vi "UI_(02)_Unlock.vi"(3 "error in (no error)":errorcluster, 4 "Settings cluster in":T1={"Defaults"={"Default User"=0.0, "VISA Resource Name "="", "Histogram parameters"={"max"=300.0, "min"=0.0, "# bins"=10, "threshold"=8.0, "thr. type"=enum."higher accepted"}}, "Recording and saving"={"Researcher name"="", "Name prefix"="", "Data post-processing"={"Filter type"=enum."Savitzky-Golay", "Length"=31, "Order"=3}, "Stop at"=0.0, "\"Stop at\" enabled"=FALSE, "Default save folder path"=path "", "Acquisition FPS"=enum."Max"}, "Geometry"={"Sensor board size"=enum."", "Bridge swap"=FALSE, "Twisted neck"=FALSE, "Bridge H. offset"=0.0, "Bridge V. offset"=0.0, "Magnets orientation"=0.0, "Cage type"=0, "Cage parameters"={"Round"=variant(i16 0), "Square"=variant(u16 0), "Donut-maze"=variant(u16 0), "T-maze"=variant(u8 0), "Sociability-maze"=variant(u8 0)}}, "IO parameters"={"IO general config."=0, "IO 1 configuration"=0, "IO 2 configuration"=0, "IO 3 configuration"=0, "IO 4 configuration"=0, "Activate ext. RS-232"=0, "IO inversion config."=0, "Sync capability"=1}, "Conditions presets array"=[{"Enabled"=FALSE, "Name"="", "Specifier(s)"=[], "Response"={"Response type"=enum."Air puff", "TTL port"=enum."Port 1", "TTL pulse length, ms"=0.0}, "Has been set"=FALSE}, {"Enabled"=FALSE, "Name"="", "Specifier(s)"=[], "Response"={"Response type"=enum."Air puff", "TTL port"=enum."Port 1", "TTL pulse length, ms"=0.0}, "Has been set"=FALSE}, {"Enabled"=FALSE, "Name"="", "Specifier(s)"=[], "Response"={"Response type"=enum."Air puff", "TTL port"=enum."Port 1", "TTL pulse length, ms"=0.0}, "Has been set"=FALSE}, {"Enabled"=FALSE, "Name"="", "Specifier(s)"=[], "Response"={"Response type"=enum."Air puff", "TTL port"=enum."Port 1", "TTL pulse length, ms"=0.0}, "Has been set"=FALSE}, {"Enabled"=FALSE, "Name"="", "Specifier(s)"=[], "Response"={"Response type"=enum."Air puff", "TTL port"=enum."Port 1", "TTL pulse length, ms"=0.0}, "Has been set"=FALSE}, {"Enabled"=FALSE, "Name"="", "Specifier(s)"=[], "Response"={"Response type"=enum."Air puff", "TTL port"=enum."Port 1", "TTL pulse length, ms"=0.0}, "Has been set"=FALSE}, {"Enabled"=FALSE, "Name"="", "Specifier(s)"=[], "Response"={"Response type"=enum."Air puff", "TTL port"=enum."Port 1", "TTL pulse length, ms"=0.0}, "Has been set"=FALSE}, {"Enabled"=FALSE, "Name"="", "Specifier(s)"=[], "Response"={"Response type"=enum."Air puff", "TTL port"=enum."Port 1", "TTL pulse length, ms"=0.0}, "Has been set"=FALSE}, {"Enabled"=FALSE, "Name"="", "Specifier(s)"=[], "Response"={"Response type"=enum."Air puff", "TTL port"=enum."Port 1", "TTL pulse length, ms"=0.0}, "Has been set"=FALSE}, {"Enabled"=FALSE, "Name"="", "Specifier(s)"=[], "Response"={"Response type"=enum."Air puff", "TTL port"=enum."Port 1", "TTL pulse length, ms"=0.0}, "Has been set"=FALSE}, {"Enabled"=FALSE, "Name"="", "Specifier(s)"=[], "Response"={"Response type"=enum."Air puff", "TTL port"=enum."Port 1", "TTL pulse length, ms"=0.0}, "Has been set"=FALSE}, {"Enabled"=FALSE, "Name"="", "Specifier(s)"=[], "Response"={"Response type"=enum."Air puff", "TTL port"=enum."Port 1", "TTL pulse length, ms"=0.0}, "Has been set"=FALSE}, {"Enabled"=FALSE, "Name"="", "Specifier(s)"=[], "Response"={"Response type"=enum."Air puff", "TTL port"=enum."Port 1", "TTL pulse length, ms"=0.0}, "Has been set"=FALSE}, {"Enabled"=FALSE, "Name"="", "Specifier(s)"=[], "Response"={"Response type"=enum."Air puff", "TTL port"=enum."Port 1", "TTL pulse length, ms"=0.0}, "Has been set"=FALSE}], "Calibration parameters"={"Timing calibration sw/hw"=1.0, "True FPS"=80.0, "True frame time, s"=80.0, "Disp. calibration info"=[]}, "Settings loaded OK"=FALSE} {"Calibration parameters"."True frame time, s" format="%.10g"; "Calibration parameters"."Disp. calibration info"."Speed, µl per ms" format="%.3g"; "Calibration parameters"."True FPS" format="%.10g"; "Calibration parameters"."Timing calibration sw/hw" format="%.10g"; "Conditions presets array"."Specifier(s)"."Validity criteria(s)"."Validity value" min=0.0 step=0.1 format="%.2g"; "Conditions presets array"."Specifier(s)"."Value" step=1.0 format="%#.2g"; "Recording and saving"."Data post-processing"."Order" min=3 max=11 step=2; "Recording and saving"."Data post-processing"."Length" min=5 max=301 step=2; "Geometry"."Cage type" items=["Round", "Square", "Donut-maze", "T-maze", "Sociability maze", ""]}, 5 "All references in":T21) -> (0 "error out":errorcluster, 1 "Settings cluster out":T1={"Defaults"={"Default User"=0.0, "VISA Resource Name "="", "Histogram parameters"={"max"=300.0, "min"=0.0, "# bins"=10, "threshold"=8.0, "thr. type"=enum."higher accepted"}}, "Recording and saving"={"Researcher name"="", "Name prefix"="", "Data post-processing"={"Filter type"=enum."Savitzky-Golay", "Length"=31, "Order"=3}, "Stop at"=0.0, "\"Stop at\" enabled"=FALSE, "Default save folder path"=path "", "Acquisition FPS"=enum."Max"}, "Geometry"={"Sensor board size"=enum."", "Bridge swap"=FALSE, "Twisted neck"=FALSE, "Bridge H. offset"=0.0, "Bridge V. offset"=0.0, "Magnets orientation"=0.0, "Cage type"=0, "Cage parameters"={"Round"=variant(i16 0), "Square"=variant(u16 0), "Donut-maze"=variant(u16 0), "T-maze"=variant(u8 0), "Sociability-maze"=variant(u8 0)}}, "IO parameters"={"IO general config."=0, "IO 1 configuration"=0, "IO 2 configuration"=0, "IO 3 configuration"=0, "IO 4 configuration"=0, "Activate ext. RS-232"=0, "IO inversion config."=0, "Sync capability"=1}, "Conditions presets array"=[{"Enabled"=FALSE, "Name"="", "Specifier(s)"=[], "Response"={"Response type"=enum."Air puff", "TTL port"=enum."Port 1", "TTL pulse length, ms"=0.0}, "Has been set"=FALSE}, {"Enabled"=FALSE, "Name"="", "Specifier(s)"=[], "Response"={"Response type"=enum."Air puff", "TTL port"=enum."Port 1", "TTL pulse length, ms"=0.0}, "Has been set"=FALSE}, {"Enabled"=FALSE, "Name"="", "Specifier(s)"=[], "Response"={"Response type"=enum."Air puff", "TTL port"=enum."Port 1", "TTL pulse length, ms"=0.0}, "Has been set"=FALSE}, {"Enabled"=FALSE, "Name"="", "Specifier(s)"=[], "Response"={"Response type"=enum."Air puff", "TTL port"=enum."Port 1", "TTL pulse length, ms"=0.0}, "Has been set"=FALSE}, {"Enabled"=FALSE, "Name"="", "Specifier(s)"=[], "Response"={"Response type"=enum."Air puff", "TTL port"=enum."Port 1", "TTL pulse length, ms"=0.0}, "Has been set"=FALSE}, {"Enabled"=FALSE, "Name"="", "Specifier(s)"=[], "Response"={"Response type"=enum."Air puff", "TTL port"=enum."Port 1", "TTL pulse length, ms"=0.0}, "Has been set"=FALSE}, {"Enabled"=FALSE, "Name"="", "Specifier(s)"=[], "Response"={"Response type"=enum."Air puff", "TTL port"=enum."Port 1", "TTL pulse length, ms"=0.0}, "Has been set"=FALSE}, {"Enabled"=FALSE, "Name"="", "Specifier(s)"=[], "Response"={"Response type"=enum."Air puff", "TTL port"=enum."Port 1", "TTL pulse length, ms"=0.0}, "Has been set"=FALSE}, {"Enabled"=FALSE, "Name"="", "Specifier(s)"=[], "Response"={"Response type"=enum."Air puff", "TTL port"=enum."Port 1", "TTL pulse length, ms"=0.0}, "Has been set"=FALSE}, {"Enabled"=FALSE, "Name"="", "Specifier(s)"=[], "Response"={"Response type"=enum."Air puff", "TTL port"=enum."Port 1", "TTL pulse length, ms"=0.0}, "Has been set"=FALSE}, {"Enabled"=FALSE, "Name"="", "Specifier(s)"=[], "Response"={"Response type"=enum."Air puff", "TTL port"=enum."Port 1", "TTL pulse length, ms"=0.0}, "Has been set"=FALSE}, {"Enabled"=FALSE, "Name"="", "Specifier(s)"=[], "Response"={"Response type"=enum."Air puff", "TTL port"=enum."Port 1", "TTL pulse length, ms"=0.0}, "Has been set"=FALSE}, {"Enabled"=FALSE, "Name"="", "Specifier(s)"=[], "Response"={"Response type"=enum."Air puff", "TTL port"=enum."Port 1", "TTL pulse length, ms"=0.0}, "Has been set"=FALSE}, {"Enabled"=FALSE, "Name"="", "Specifier(s)"=[], "Response"={"Response type"=enum."Air puff", "TTL port"=enum."Port 1", "TTL pulse length, ms"=0.0}, "Has been set"=FALSE}], "Calibration parameters"={"Timing calibration sw/hw"=1.0, "True FPS"=80.0, "True frame time, s"=80.0, "Disp. calibration info"=[]}, "Settings loaded OK"=FALSE} {"Calibration parameters"."True frame time, s" format="%.10g"; "Calibration parameters"."Disp. calibration info"."Speed, µl per ms" format="%.3g"; "Calibration parameters"."True FPS" format="%.10g"; "Calibration parameters"."Timing calibration sw/hw" format="%.10g"; "Conditions presets array"."Specifier(s)"."Validity criteria(s)"."Validity value" min=0.0 step=0.1 format="%.2g"; "Conditions presets array"."Specifier(s)"."Value" step=1.0 format="%#.2g"; "Recording and saving"."Data post-processing"."Order" min=3 max=11 step=2; "Recording and saving"."Data post-processing"."Length" min=5 max=301 step=2; "Geometry"."Cage type" items=["Round", "Square", "Donut-maze", "T-maze", "Sociability maze", ""]}, 2 "All references out":T21)   [LabVIEW 2018, in "Tracker.lvlib"]
uses:
  Tracker.lvlib
  Controls/CTL_All_References.ctl
  Controls/CTL_Controls_References.ctl
  Controls/CTL_Indicators_References.ctl
  Common/Typedefs/CTL_Panes_and_VIs_References.ctl
  Controls/CTL_Histogram_Properties.ctl
  <vilib>/Utility/miscctls.llb/LVRangeTypeDef.ctl
  Controls/CTL_Settings_cluster.ctl
  Controls/CTL_Histogram_parameters.ctl
  Controls/CTL_Filter_selector.ctl
  Controls/CTL_Acquisition_speed_selector.ctl
  Common/Typedefs/CTL_Segmented_plot_parameters_2.ctl
  Libraries/Cage Diagram/Typedefs/CTL_Cage_type.ctl
  Controls/CTL_Cage_all_segmentation_params_set.ctl
  Controls/CTL_IO_params_cluster.ctl
  Controls/CTL_Conditions_Array.ctl
  Controls/CTL_Conditions_Cluster.ctl
  Controls/CTL_Condition_type.ctl
  Controls/CTL_Comparison_type.ctl
  Controls/CTL_Validity_check_criteria.ctl
  Controls/CTL_Response_info.ctl
  Controls/CTL_Condition_response_type.ctl
  Controls/CTL_Reponse_port_info.ctl
  Controls/CTL_Calibration_parameters.ctl
  Controls/CTL_Dispenser_calibration_info.ctl
  Common/Typedefs/CTL_Segmented_plot_parameters_2_(round_d1).ctl
  <vilib>/Utility/error.llb/Error Cluster From Error Code.vi
  <vilib>/ErrorRing/Error Ring.xnode
  Common_Resources.lvlib
  Libraries/Cage Diagram/Cage Diagram.lvlib
panel:
  in  "Histogram initialization cluster":T19={"X Scale.Range"={"Minimum"=0.0, "Maximum"=13.0, "Increment"=1.0, "Minor Increment"=1.0, "Start"=0.0}, "Caption.Text"="Zone preference (normalized)", "X Scale.Offset and Multiplier:Multiplier"=1.0, "X Scale.Offset and Multiplier:Offset"=0.0, "X Scale.Scale Fit"=2, "X Scale.Display Format:Precision"=0, "Y Scale.Mapping Mode"=0, "Zones preference empty initialized array"=[0, 0, 0, 0, 0, 0, 0, 0, 0, 0, 0, 0, 0, 0], "Plot.Fill/Point Color"=15790320}
  out "Panes references":T24
  out "Controls references params":string[][](array[string])
  out "Indicators references params":string[][](array[string])
  out "Indicators references":T23
  out "Controls references":T22
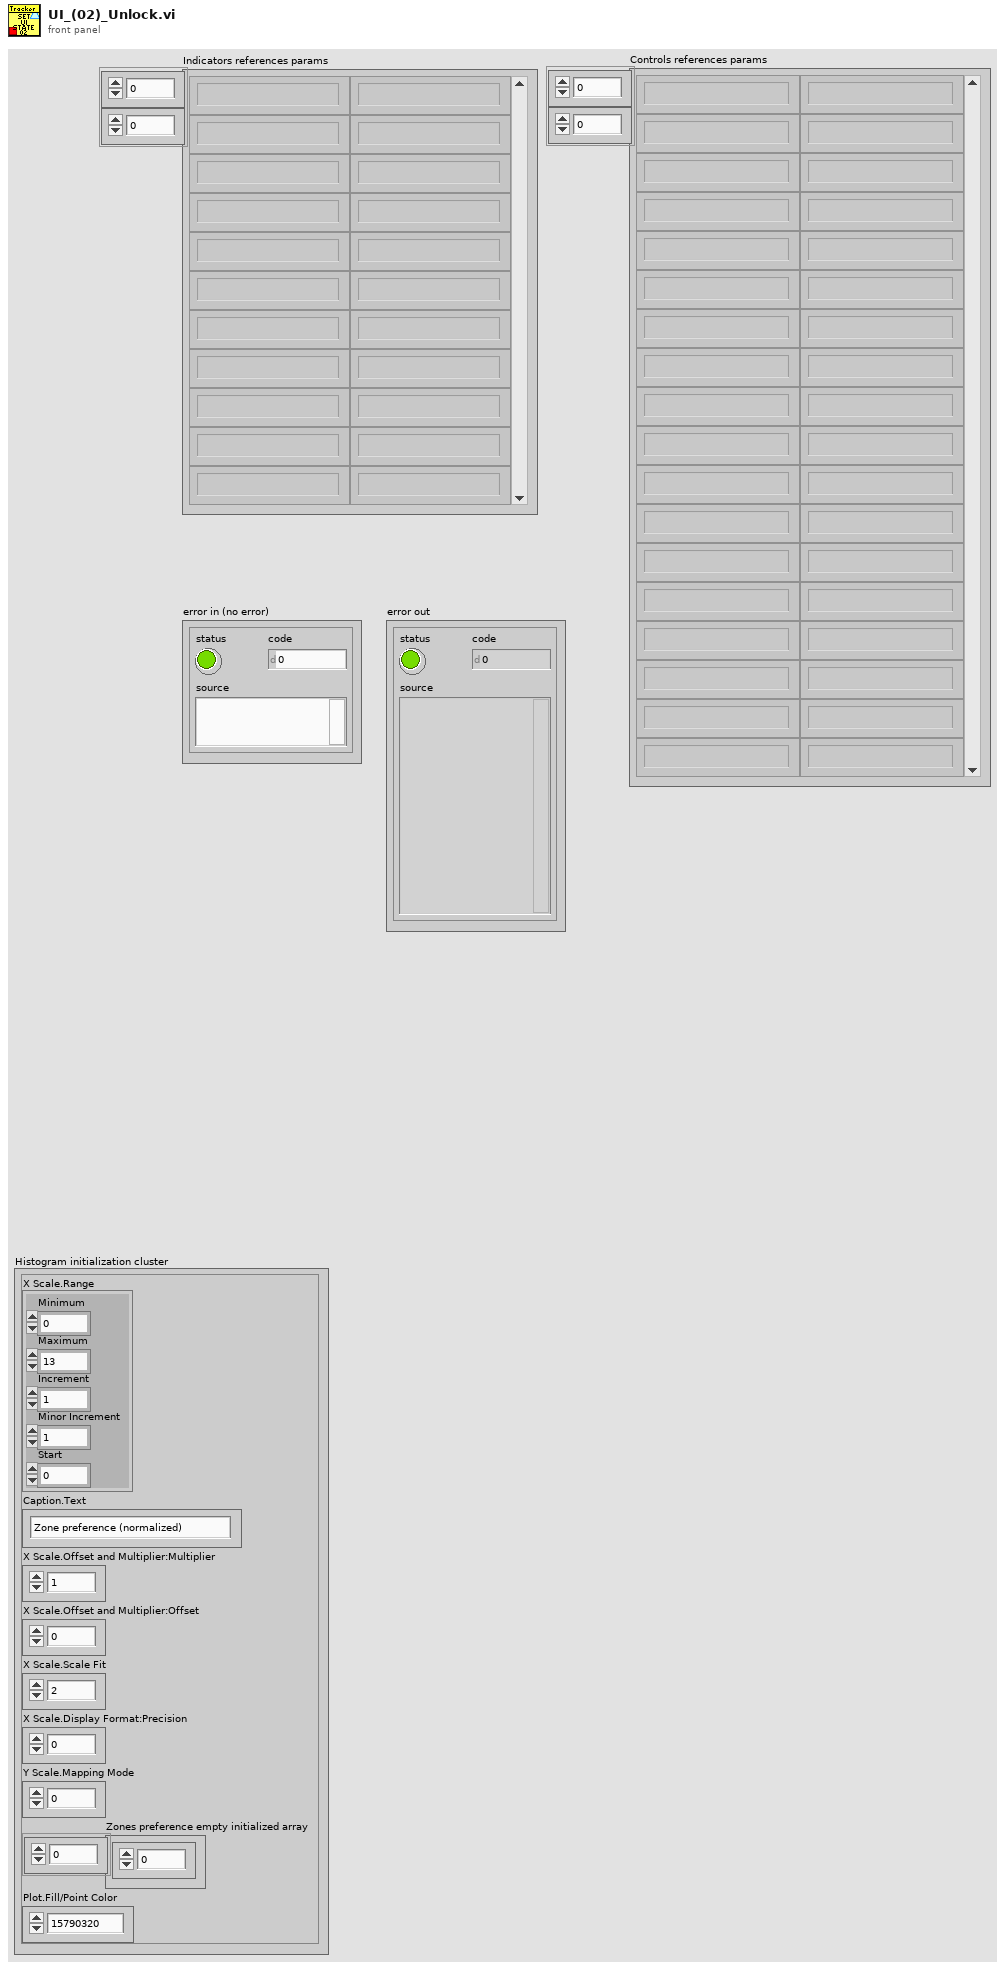
[diagram p1: front panel]
types:
  T1 = typedef "Common_Resources.lvlib/CTL_Settings_cluster.ctl" = cluster{"Defaults":cluster{"Default User":dbl, "VISA Resource Name ":string, "Histogram parameters":T2}, "Recording and saving":cluster{"Researcher name":string, "Name prefix":string, "Data post-processing":T3, "Stop at":dbl, "\"Stop at\" enabled":bool, "Default save folder path":path, "Acquisition FPS":T4}, "Geometry":T5, "IO parameters":T8, "Conditions presets array":T9, "Calibration parameters":T17, "Settings loaded OK":bool}
  T2 = typedef "Common_Resources.lvlib/CTL_Histogram_parameters.ctl" = cluster{"max":dbl, "min":dbl, "# bins":i32, "threshold":dbl, "thr. type":enum16{"higher accepted", "lower accepted"}}
  T3 = typedef "Common_Resources.lvlib/CTL_Filter_selector.ctl" = cluster{"Filter type":enum16{"None", "Savitzky-Golay"}, "Length":i32, "Order":i32}
  T4 = typedef "Common_Resources.lvlib/CTL_Acquisition_speed_selector.ctl" = enum16{"Max", "Optimal", "Eco"}
  T5 = typedef "Common_Resources.lvlib/CTL_Segmented_plot_parameters_2.ctl" = cluster{"Sensor board size":enum16{"", "Large"}, "Bridge swap":bool, "Twisted neck":bool, "Bridge H. offset":sgl, "Bridge V. offset":sgl, "Magnets orientation":sgl, "Cage type":T6, "Cage parameters":T7}
  T6 = typedef "Cage Diagram.lvlib/CTL_Cage_type.ctl" = u16
  T7 = typedef "Common_Resources.lvlib/CTL_Cage_all_segmentation_params_set.ctl" = cluster{"Round":variant, "Square":variant, "Donut-maze":variant, "T-maze":variant, "Sociability-maze":variant}
  T8 = typedef "Common_Resources.lvlib/CTL_IO_params_cluster.ctl" = cluster{"IO general config.":u16, "IO 1 configuration":u16, "IO 2 configuration":u16, "IO 3 configuration":u16, "IO 4 configuration":u16, "Activate ext. RS-232":u16, "IO inversion config.":u16, "Sync capability":u8}
  T9 = typedef "Common_Resources.lvlib/CTL_Conditions_Array.ctl" = T10[]
  T10 = typedef "Common_Resources.lvlib/CTL_Conditions_Cluster.ctl" = cluster{"Enabled":bool, "Name":string, "Specifier(s)":cluster{"Specifier enabled":bool, "Condition type":T11, "Comparison type":T12, "Value":dbl, "Validity criteria(s)":cluster{"V. check enabled":bool, "Criteria":T13, "Validity value":dbl}[]}[], "Response":T14, "Has been set":bool}
  T11 = typedef "Common_Resources.lvlib/CTL_Condition_type.ctl" = enum16{"Speed", "Zone", "Angle to wall"}
  T12 = typedef "Common_Resources.lvlib/CTL_Comparison_type.ctl" = enum16{"Less", "Less or Equal", "Equal", "Greater or Equal", "Greater", "Not Equal"}
  T13 = typedef "Common_Resources.lvlib/CTL_Validity_check_criteria.ctl" = enum16{"Running bout (seconds)", "Running bout (meters)"}
  T14 = typedef "Common_Resources.lvlib/CTL_Response_info.ctl" = cluster{"Response type":T15, "TTL port":T16, "TTL pulse length, ms":dbl}
  T15 = typedef "Common_Resources.lvlib/CTL_Condition_response_type.ctl" = enum16{"None", "Air puff", "Liquid reward", "TTL pulse", "TTL pulse (ubr)", "TTL signal"}
  T16 = typedef "Common_Resources.lvlib/CTL_Reponse_port_info.ctl" = enum16{"Port 1", "Port 2", "Port 3", "Port 4"}
  T17 = typedef "Common_Resources.lvlib/CTL_Calibration_parameters.ctl" = cluster{"Timing calibration sw/hw":dbl, "True FPS":dbl, "True frame time, s":dbl, "Disp. calibration info":T18}
  T18 = typedef "Common_Resources.lvlib/CTL_Dispenser_calibration_info.ctl" = cluster{"Channel":u8, "Speed, µl per ms":dbl}[]
  T19 = typedef "Common_Resources.lvlib/CTL_Histogram_Properties.ctl" = cluster{"X Scale.Range":T20, "Caption.Text":string, "X Scale.Offset and Multiplier:Multiplier":dbl, "X Scale.Offset and Multiplier:Offset":dbl, "X Scale.Scale Fit":u8, "X Scale.Display Format:Precision":u8, "Y Scale.Mapping Mode":u8, "Zones preference empty initialized array":i32[], "Plot.Fill/Point Color":u32}
  T20 = typedef "LVRangeTypeDef.ctl" = cluster{"Minimum":dbl, "Maximum":dbl, "Increment":dbl, "Minor Increment":dbl, "Start":dbl}
  T21 = typedef "Common_Resources.lvlib/CTL_All_References.ctl" = cluster{"Controls references":T22, "Indicators references":T23, "Service references":T24}
  T22 = typedef "Common_Resources.lvlib/CTL_Controls_References.ctl" = cluster{"Check HW connection":refnum<vi>, "Save settings":refnum<vi>, "Reset zones":refnum<vi>, "Reset stimuli":refnum<vi>, "Record/Stop":refnum<vi>, "Reset barplot":refnum<vi>, "Multiplyer of chart RX":refnum<vi>, "Show zones":refnum<vi>, "Show magnets":refnum<vi>, "Show heatmap":refnum<vi>, "Show full track":refnum<vi>, "Open File":refnum<vi>, "Play/Pause":refnum<vi>, "Trace, s":refnum<vi>, "Playback speed":refnum<vi>, "Timeline":refnum<vi>, "By Zone stim. setup":refnum<vi>, "Set/Rec and Analyse Tab":refnum<vi>, "Cage radial segmentation":refnum<vi>, "Set IO config":refnum<vi>, "Rainbow (time)":refnum<vi>, "Rainbow (speed)":refnum<vi>, "Add Reward":refnum<vi>, "Modify Reward":refnum<vi>, "Delete Reward":refnum<vi>, "Speed threshold, mm/s":refnum<vi>, "Start Over":refnum<vi>}
  T23 = typedef "Common_Resources.lvlib/CTL_Indicators_References.ctl" = cluster{"HW info":refnum<vi>, "Port":refnum<vi>, "Ready":refnum<vi>, "IO status indicator":refnum<vi>, "Current Time":refnum<vi>, "Record timestamp":refnum<vi>, "Mouse speed":refnum<vi>, "Mouse speed, mm/s":refnum<vi>, "Running, perc. of time":refnum<vi>, "Histograms":refnum<vi>, "Cage size":refnum<vi>, "Reward":refnum<vi>, "Current zone":refnum<vi>, "Run length, m":refnum<vi>}
  T24 = typedef "Common_Resources.lvlib/CTL_Panes_and_VIs_References.ctl" = cluster{"Pane":refnum<vi>, "This VI":refnum<vi>, "Menu":refnum<k9>}
  T25 = typedef "Common_Resources.lvlib/CTL_Segmented_plot_parameters_2_(round_d1).ctl" = cluster{"Cage diameter, mm":u16, "Starting angle BORDER":i16, "Starting angle MIDFIELD":i16, "Radius, mm MIDFIELD":u16, "Radius, mm CENTER":u16, "N segments BORDER":u8, "N segments MIDFIELD":u8, "R-gap, mm":sgl}
  T26 = enum8{"Enabled", "Disabled", "Disabled and Grayed Out"}
  T27 = enum32{"Page Enabled", "Page Disabled", "Page Disabled & Grayed"}
  T28 = cluster{"Slider":dbl, "Slider":dbl, "Slider":dbl}
  T29 = cluster{"Radius, mm MIDFIELD":u16, "N segments MIDFIELD":u8, "Starting angle MIDFIELD":i16}
  T30 = cluster{"N segments BORDER":u8, "Starting angle BORDER":i16}
  T31 = cluster{cluster{"Radius, mm CENTER":u16}, cluster{"Radius, mm MIDFIELD":u16, "N segments MIDFIELD":u8, "Starting angle MIDFIELD":i16}, cluster{"N segments BORDER":u8, "Starting angle BORDER":i16}}
  T32 = typedef "Common_Resources.lvlib/CTL_IO_status_indicator.ctl" = cluster{"IO1":bool, "IO2":bool, "IO3":bool, "IO4":bool, "St1":bool, "St2":bool, "St3":bool, "St4":bool, "Z1":bool, "Z2":bool, "Z3":bool, "Z4":bool, "Syn1":bool, "Syn2":bool, "RS-232 ext. activated":bool}
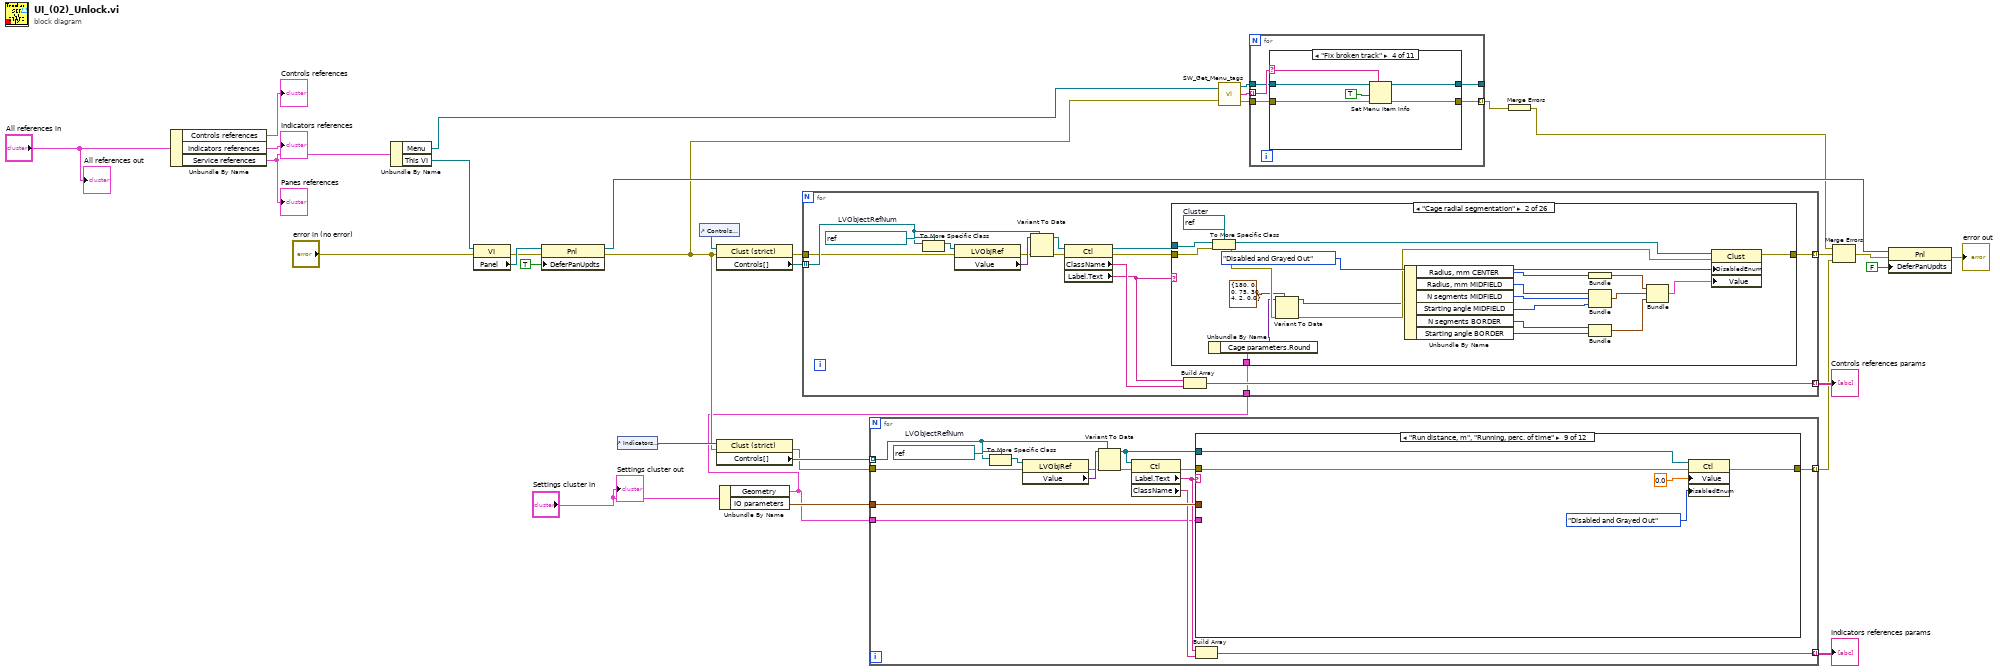
[diagram p0: block diagram]
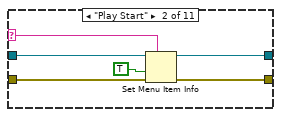
[diagram p3: hidden frame]
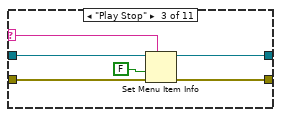
[diagram p4: hidden frame]
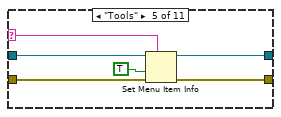
[diagram p5: hidden frame]
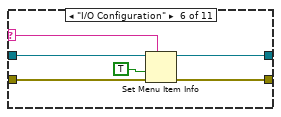
[diagram p6: hidden frame]
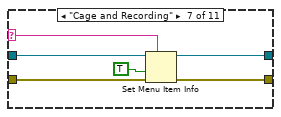
[diagram p7: hidden frame]
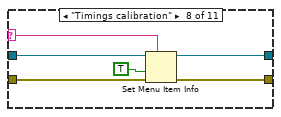
[diagram p8: hidden frame]
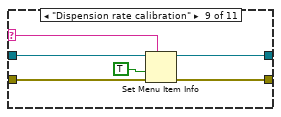
[diagram p9: hidden frame]
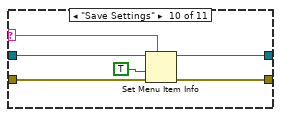
[diagram p10: hidden frame]
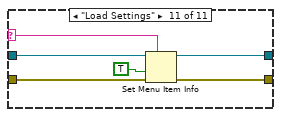
[diagram p11: hidden frame]
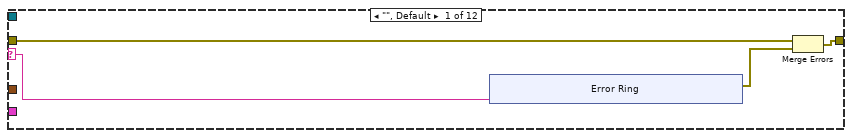
[diagram p12: hidden frame]
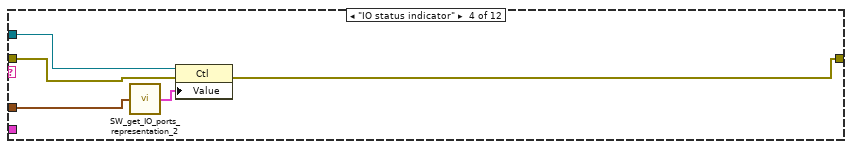
[diagram p15: hidden frame]
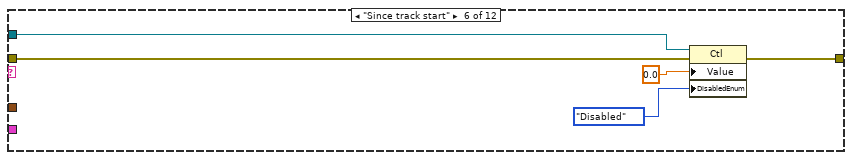
[diagram p17: hidden frame]
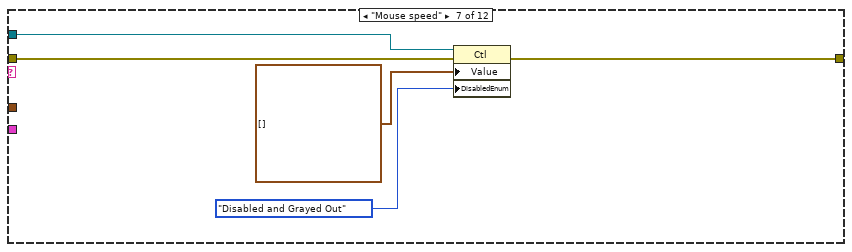
[diagram p18: hidden frame]
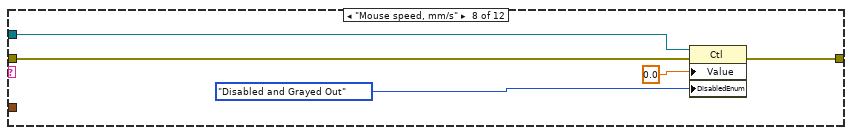
[diagram p19: hidden frame]
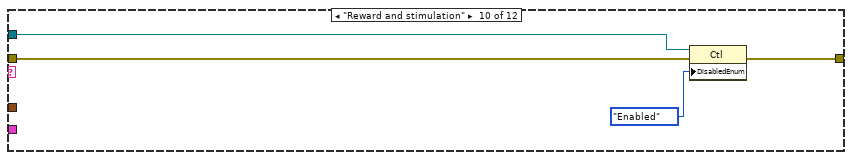
[diagram p20: hidden frame]
diagram:
  n1 = Unbundle By Name("All references in") -> ("Controls references"=→"Controls references":T22, "Indicators references"=→"Indicators references":T23, "Service references"=w24:T24)
  "Panes references" <- w24
  n2 = Unbundle By Name(w24) -> ("Menu"=w4:refnum<k9>, "This VI"=w21:refnum<vi>)
  n3 = property class="VI"(reference=w21, error in="error in (no error)") -> (error out=w14:errorcluster, "Panel"=w23:refnum<vi>)  [unwired: 1 out]
  n4 = property class="Pnl"(reference=w23, error in=w14, "DeferPanUpdts"=TRUE ("Defer Panel Updates")) -> (reference out=w15:refnum<vi>, error out=w3:errorcluster)
  n5 = control-ref of="Indicators references"() -> (w27:refnum<vi>)
  n6 = control-ref of="Controls references"() -> (w29:refnum<vi>)
  n7 = property class="Clust (strict)"(reference=w29, error in=w3) -> (error out=w20:errorcluster, "Controls[]"=w30:refnum<vi>[])  [unwired: 1 out]
  n8 = property class="Clust (strict)"(reference=w27, error in=w3) -> (error out=w19:errorcluster, "Controls[]"=w28:refnum<vi>[])  [unwired: 1 out]
  n9 = Unbundle By Name("Settings cluster in") -> ("Geometry"=w1:T5, "IO parameters"=w10:T8)
  n10 = for {
    tunnel: w30 -> [w45] mode=indexing
    tunnel: [w42] -> w25 mode=indexing
    tunnel: w20 -> [w41]
    tunnel: [w37] -> w12 mode=indexing
    tunnel: w1 -> [w34]
    w47 = refnum<vi> refnum  # LVObjectRefNum
    n11 = To More Specific Class(target class=w47, reference=w45) -> (specific class reference=w48:refnum<vi>)  [unwired: 1 in, 1 out]
    n12 = property class="LVObjRef"(reference=w48, error in=w41) -> (error out=w40:errorcluster, "Value"=w46:variant)  [unwired: 1 out]
    n13 = Variant To Data(error in=w40, type=w45, Variant=w46) -> (data=w44:refnum<vi>, error out=w39:errorcluster)
    n14 = property class="Ctl"(reference=w44, error in=w39) -> (reference out=w35:refnum<vi>, error out=w36:errorcluster, "ClassName"=w43:string, "Label.Text"=w38:string)
    n15 = case shown="\"Cage radial segmentation\"" w38 {
      selector: w38 -> [w49 _ _ _ _ _ _ _ _ _ _ _ _ _ _ _ _ _ _ _ _ _ _ _ _ _]
      tunnel: [w51 w80 w82 w98 w106 w114 w122 w130 w139 w148 w156 w164 w172 w180 w188 w196 w204 w212 w220 w228 w236 w244 w251 w259 w271 w278] -> w37
      tunnel: w36 -> [w52 w81 w83 w100 w108 w116 w124 w132 w141 w150 w158 w166 w174 w182 w190 w198 w206 w214 w222 w230 w238 w246 w253 w261 w273 w280]
      tunnel: w35 -> [_ w68 w84 w103 w111 w119 w127 w135 w144 w153 w161 w169 w177 w185 w193 w201 w209 w217 w225 w233 w241 w249 w256 w264 w276 w283]
      tunnel: w34 -> [_ w62 _ _ _ _ _ _ _ _ _ _ _ _ _ _ _ _ _ _ _ _ _ _ _ _]
      frame "", Default {
        n16 = xnode "Error Ring"("parameter 0"=w49) -> ("error out"=w50:errorcluster)
        n17 = Merge Errors(w52, w50) -> (w51:errorcluster)
      }
      frame "Cage radial segmentation" {
        w66 = refnum<vi> refnum  # Cluster
        n18 = Unbundle By Name(w62) -> ("Cage parameters.Round"=w61:variant)
        n19 = To More Specific Class(target class=w66, reference=w68, error in=w81) -> (specific class reference=w67:refnum<vi>, error out=w65:errorcluster)
        n20 = Variant To Data(error in=w65, type=T25 {"Cage diameter, mm"=180, "Starting angle BORDER"=0, "Starting angle MIDFIELD"=0, "Radius, mm MIDFIELD"=75, "Radius, mm CENTER"=30, "N segments BORDER"=4, "N segments MIDFIELD"=2, "R-gap, mm"=0.0} ("Radial segmentation parameters"), Variant=w61) -> (data=w60:T25, error out=w64:errorcluster)
        n21 = Unbundle By Name(w60) -> ("Radius, mm CENTER"=w78:u16, "Radius, mm MIDFIELD"=w77:u16, "N segments MIDFIELD"=w76:u8, "Starting angle MIDFIELD"=w75:i16, "N segments BORDER"=w74:u8, "Starting angle BORDER"=w73:i16)
        n22 = Bundle("Radius, mm CENTER"=w78) -> (w72:cluster{"Radius, mm CENTER":u16})  [unwired: 1 in]
        n23 = Bundle("Radius, mm MIDFIELD"=w77, "N segments MIDFIELD"=w76, "Starting angle MIDFIELD"=w75) -> (w71:T29)  [unwired: 1 in]
        n24 = Bundle("N segments BORDER"=w74, "Starting angle BORDER"=w73) -> (w70:T30)  [unwired: 1 in]
        n25 = Bundle(w72, w71, w70) -> (w69:T31)  [unwired: 1 in]
        n26 = property class="Clust"(reference=w67, error in=w64, "DisabledEnum"=T26."Disabled and Grayed Out" ("Disabled"), "Value"=w69) -> (error out=w80:errorcluster)  [unwired: 1 out]
      }
      frame "Set/Rec and Analyse Tab" {
        w89 = refnum<vi> refnum  # TabControl
        n27 = To More Specific Class(target class=w89, reference=w84, error in=w83) -> (specific class reference=w90:refnum<vi>, error out=w87:errorcluster)
        n28 = property class="TabCtl"(reference=w90, error in=w87, "Value"=enum32{"Settings", "Recording and Analysis"}."Settings") -> (error out=w86:errorcluster, "Pages"=w88:refnum<vi>[])  [unwired: 1 out]
        n29 = for {
          tunnel: w88 -> [w94] mode=indexing
          tunnel: w86 -> [w93]
          tunnel: [w92] -> w85 mode=indexing
          n30 = property class="Page"(reference=w94, error in=w93, "PageEnb"=T27."Page Enabled" ("Page Enabled State")) -> (error out=w92:errorcluster)  [unwired: 1 out]
        }
        n31 = Merge Errors(w85) -> (w82:errorcluster)
      }
      frame "Check HW connection" {
        w102 = refnum<vi> refnum  # Boolean
        n32 = To More Specific Class(target class=w102, reference=w103, error in=w100) -> (specific class reference=w101:refnum<vi>, error out=w99:errorcluster)
        n33 = property class="Bool"(reference=w101, error in=w99, "Value"=FALSE, "DisabledEnum"=T26."Disabled and Grayed Out" ("Disabled")) -> (error out=w98:errorcluster)  [unwired: 1 out]
      }
      frame "Save settings" {
        w110 = refnum<vi> refnum  # Boolean
        n34 = To More Specific Class(target class=w110, reference=w111, error in=w108) -> (specific class reference=w109:refnum<vi>, error out=w107:errorcluster)
        n35 = property class="Bool"(reference=w109, error in=w107, "Value"=FALSE, "DisabledEnum"=T26."Enabled" ("Disabled")) -> (error out=w106:errorcluster)  [unwired: 1 out]
      }
      frame "Set IO config" {
        w118 = refnum<vi> refnum  # Boolean
        n36 = To More Specific Class(target class=w118, reference=w119, error in=w116) -> (specific class reference=w117:refnum<vi>, error out=w115:errorcluster)
        n37 = property class="Bool"(reference=w117, error in=w115, "Value"=FALSE, "DisabledEnum"=T26."Enabled" ("Disabled")) -> (error out=w114:errorcluster)  [unwired: 1 out]
      }
      frame "Reset zones" {
        w126 = refnum<vi> refnum  # Boolean
        n38 = To More Specific Class(target class=w126, reference=w127, error in=w124) -> (specific class reference=w125:refnum<vi>, error out=w123:errorcluster)
        n39 = property class="Bool"(reference=w125, error in=w123, "Value"=FALSE, "DisabledEnum"=T26."Enabled" ("Disabled")) -> (error out=w122:errorcluster)  [unwired: 1 out]
      }
      frame "Reset stimuli" {
        w134 = refnum<vi> refnum  # Boolean
        n40 = To More Specific Class(target class=w134, reference=w135, error in=w132) -> (specific class reference=w133:refnum<vi>, error out=w131:errorcluster)
        n41 = property class="Bool"(reference=w133, error in=w131, "Value"=FALSE, "DisabledEnum"=T26."Enabled" ("Disabled")) -> (error out=w130:errorcluster)  [unwired: 1 out]
      }
      frame "Record/Stop" {
        w143 = refnum<vi> refnum  # Boolean
        n42 = To More Specific Class(target class=w143, reference=w144, error in=w141) -> (specific class reference=w142:refnum<vi>, error out=w140:errorcluster)
        n43 = property class="Bool"(reference=w142, error in=w140, "Value"=FALSE, "DisabledEnum"=T26."Disabled and Grayed Out" ("Disabled"), "Visible"=TRUE) -> (error out=w139:errorcluster)  [unwired: 1 out]
      }
      frame "Start over" {
        w152 = refnum<vi> refnum  # Boolean
        n44 = To More Specific Class(target class=w152, reference=w153, error in=w150) -> (specific class reference=w151:refnum<vi>, error out=w149:errorcluster)
        n45 = property class="Bool"(reference=w151, error in=w149, "Value"=FALSE, "DisabledEnum"=T26."Disabled and Grayed Out" ("Disabled"), "Visible"=FALSE) -> (error out=w148:errorcluster)  [unwired: 1 out]
      }
      frame "Reset barplot" {
        w160 = refnum<vi> refnum  # Boolean
        n46 = To More Specific Class(target class=w160, reference=w161, error in=w158) -> (specific class reference=w159:refnum<vi>, error out=w157:errorcluster)
        n47 = property class="Bool"(reference=w159, error in=w157, "Value"=FALSE, "DisabledEnum"=T26."Disabled and Grayed Out" ("Disabled")) -> (error out=w156:errorcluster)  [unwired: 1 out]
      }
      frame "Multiplyer of chart RX" {
        w168 = refnum<vi> refnum  # Slide
        n48 = To More Specific Class(target class=w168, reference=w169, error in=w166) -> (specific class reference=w167:refnum<vi>, error out=w165:errorcluster)
        n49 = property class="Slide"(reference=w167, error in=w165, "Value"=u8 1, "DisabledEnum"=T26."Disabled and Grayed Out" ("Disabled")) -> (error out=w164:errorcluster)  [unwired: 1 out]
      }
      frame "Show zones" {
        w176 = refnum<vi> refnum  # Boolean
        n50 = To More Specific Class(target class=w176, reference=w177, error in=w174) -> (specific class reference=w175:refnum<vi>, error out=w173:errorcluster)
        n51 = property class="Bool"(reference=w175, error in=w173, "Value"=TRUE, "DisabledEnum"=T26."Enabled" ("Disabled")) -> (error out=w172:errorcluster)  [unwired: 1 out]
      }
      frame "Show magnets" {
        w184 = refnum<vi> refnum  # Boolean
        n52 = To More Specific Class(target class=w184, reference=w185, error in=w182) -> (specific class reference=w183:refnum<vi>, error out=w181:errorcluster)
        n53 = property class="Bool"(reference=w183, error in=w181, "Value"=TRUE, "DisabledEnum"=T26."Disabled and Grayed Out" ("Disabled")) -> (error out=w180:errorcluster)  [unwired: 1 out]
      }
      frame "Rainbow (speed)", "Rainbow (time)" {
        w192 = refnum<vi> refnum  # Boolean
        n54 = To More Specific Class(target class=w192, reference=w193, error in=w190) -> (specific class reference=w191:refnum<vi>, error out=w189:errorcluster)
        n55 = property class="Bool"(reference=w191, error in=w189, "Value"=FALSE, "DisabledEnum"=T26."Disabled and Grayed Out" ("Disabled")) -> (error out=w188:errorcluster)  [unwired: 1 out]
      }
      frame "Add Reward" {
        w200 = refnum<vi> refnum  # Boolean
        n56 = To More Specific Class(target class=w200, reference=w201, error in=w198) -> (specific class reference=w199:refnum<vi>, error out=w197:errorcluster)
        n57 = property class="Bool"(reference=w199, error in=w197, "Value"=FALSE, "DisabledEnum"=T26."Disabled and Grayed Out" ("Disabled")) -> (error out=w196:errorcluster)  [unwired: 1 out]
      }
      frame "Modify Reward", "Remove Reward" {
        w208 = refnum<vi> refnum  # Boolean
        n58 = To More Specific Class(target class=w208, reference=w209, error in=w206) -> (specific class reference=w207:refnum<vi>, error out=w205:errorcluster)
        n59 = property class="Bool"(reference=w207, error in=w205, "Value"=FALSE, "DisabledEnum"=T26."Disabled and Grayed Out" ("Disabled")) -> (error out=w204:errorcluster)  [unwired: 1 out]
      }
      frame "Show heatmap" {
        w216 = refnum<vi> refnum  # Boolean
        n60 = To More Specific Class(target class=w216, reference=w217, error in=w214) -> (specific class reference=w215:refnum<vi>, error out=w213:errorcluster)
        n61 = property class="Bool"(reference=w215, error in=w213, "Value"=FALSE, "DisabledEnum"=T26."Disabled and Grayed Out" ("Disabled")) -> (error out=w212:errorcluster)  [unwired: 1 out]
      }
      frame "Show full track" {
        w224 = refnum<vi> refnum  # Boolean
        n62 = To More Specific Class(target class=w224, reference=w225, error in=w222) -> (specific class reference=w223:refnum<vi>, error out=w221:errorcluster)
        n63 = property class="Bool"(reference=w223, error in=w221, "Value"=FALSE, "DisabledEnum"=T26."Disabled and Grayed Out" ("Disabled")) -> (error out=w220:errorcluster)  [unwired: 1 out]
      }
      frame "Open File" {
        w232 = refnum<vi> refnum  # Boolean
        n64 = To More Specific Class(target class=w232, reference=w233, error in=w230) -> (specific class reference=w231:refnum<vi>, error out=w229:errorcluster)
        n65 = property class="Bool"(reference=w231, error in=w229, "Value"=FALSE, "DisabledEnum"=T26."Enabled" ("Disabled")) -> (error out=w228:errorcluster)  [unwired: 1 out]
      }
      frame "Play/Pause" {
        w240 = refnum<vi> refnum  # Boolean
        n66 = To More Specific Class(target class=w240, reference=w241, error in=w238) -> (specific class reference=w239:refnum<vi>, error out=w237:errorcluster)
        n67 = property class="Bool"(reference=w239, error in=w237, "Value"=FALSE, "DisabledEnum"=T26."Enabled" ("Disabled")) -> (error out=w236:errorcluster)  [unwired: 1 out]
      }
      frame "Trace, s" {
        w248 = refnum<vi> refnum  # Slide
        n68 = To More Specific Class(target class=w248, reference=w249, error in=w246) -> (specific class reference=w247:refnum<vi>, error out=w245:errorcluster)
        n69 = property class="Slide"(reference=w247, error in=w245, "Value"=u8 5, "DisabledEnum"=T26."Disabled and Grayed Out" ("Disabled")) -> (error out=w244:errorcluster)  [unwired: 1 out]
      }
      frame "Speed threshold" {
        w255 = refnum<vi> refnum  # Digital
        n70 = To More Specific Class(target class=w255, reference=w256, error in=w253) -> (specific class reference=w254:refnum<vi>, error out=w252:errorcluster)
        n71 = property class="DigNum"(reference=w254, error in=w252, "DisabledEnum"=T26."Disabled and Grayed Out" ("Disabled")) -> (error out=w251:errorcluster)  [unwired: 1 out]
      }
      frame "Playback speed" {
        w263 = refnum<vi> refnum  # Ring
        n72 = To More Specific Class(target class=w263, reference=w264, error in=w261) -> (specific class reference=w262:refnum<vi>, error out=w260:errorcluster)
        n73 = property class="Ring"(reference=w262, error in=w260, "Value"=u8 120, "DisabledEnum"=T26."Disabled and Grayed Out" ("Disabled")) -> (error out=w259:errorcluster)  [unwired: 1 out]
      }
      frame "Timeline" {
        w265 = 0.0 ("Slider")
        w275 = refnum<vi> refnum  # Slide
        n74 = To More Specific Class(target class=w275, reference=w276, error in=w273) -> (specific class reference=w274:refnum<vi>, error out=w272:errorcluster)
        n75 = Bundle(cluster=T28 {"Slider"=0.0, "Slider"=0.0, "Slider"=0.0} ("Timeline"), "Slider"=w265, "Slider"=0.001, "Slider"=w265) -> (w268:T28)
        n76 = To Variant(anything=w268) -> (Variant=w267:variant)
        n77 = property class="Slide"(reference=w274, error in=w272, "Value"=w267, "DisabledEnum"=T26."Disabled and Grayed Out" ("Disabled")) -> (error out=w271:errorcluster)  [unwired: 1 out]
      }
      frame "By Zone stim. setup" {
        w282 = refnum<vi> refnum  # RadioButtonsControl
        n78 = To More Specific Class(target class=w282, reference=w283, error in=w280) -> (specific class reference=w281:refnum<vi>, error out=w279:errorcluster)
        n79 = property class="RadioBtnsControl"(reference=w281, error in=w279, "DisabledEnum"=T26."Enabled" ("Disabled")) -> (error out=w278:errorcluster)  [unwired: 1 out]
      }
    }
    n80 = Build Array(w38, w43) -> (w42:string[])
  }
  "Controls references params" <- w25
  n81 = for {
    tunnel: w28 -> [w295] mode=indexing
    tunnel: [w285] -> w26 mode=indexing
    tunnel: w19 -> [w293]
    tunnel: [w289] -> w18 mode=indexing
    tunnel: w10 -> [w288]
    tunnel: w1 -> [w284]
    w297 = refnum<vi> refnum  # LVObjectRefNum
    n82 = To More Specific Class(target class=w297, reference=w295) -> (specific class reference=w298:refnum<vi>)  [unwired: 1 in, 1 out]
    n83 = property class="LVObjRef"(reference=w298, error in=w293) -> (error out=w292:errorcluster, "Value"=w296:variant)  [unwired: 1 out]
    n84 = Variant To Data(error in=w292, type=w295, Variant=w296) -> (data=w294:refnum<vi>, error out=w291:errorcluster)
    n85 = property class="Ctl"(reference=w294, error in=w291) -> (error out=w290:errorcluster, "Label.Text"=w287:string, "ClassName"=w286:string)  [unwired: 1 out]
    n86 = case shown="\"Run distance, m\", \"Running, perc. of time\"" w287 {
      selector: w287 -> [w299 _ _ _ _ _ _ _ _ _ _ _]
      tunnel: w294 -> [_ _ _ w313 _ w322 w327 w332 w337 w341 w348 w350]
      tunnel: w290 -> [w302 w310 w311 w314 w317 w321 w326 w331 w336 w340 w344 w352]
      tunnel: [w301 w310 w311 w316 w317 w320 w325 w330 w335 w339 w347 w349] -> w289
      tunnel: w288 -> [_ _ _ w315 _ _ _ _ _ _ _ _]
      tunnel: w284 -> [_ _ _ _ _ _ _ _ _ _ _ w351]
      frame "", Default {
        n87 = xnode "Error Ring"("parameter 0"=w299) -> ("error out"=w300:errorcluster)
        n88 = Merge Errors(w302, w300) -> (w301:errorcluster)
      }
      frame "Cage size", "HW info", "Port" {
      }
      frame "Ready" {
      }
      frame "IO status indicator" {
        n89 = call "SW_get_IO_ports_representation_2.vi"("Sync parameters cluster input"=w315) -> ("IO status indicator"=w312:T32)
        n90 = property class="Ctl"(reference=w313, error in=w314, "Value"=w312) -> (error out=w316:errorcluster)  [unwired: 1 out]
      }
      frame "Current Time" {
      }
      frame "Since track start" {
        n91 = property class="Ctl"(reference=w322, error in=w321, "Value"=0.0, "DisabledEnum"=T26."Disabled" ("Disabled")) -> (error out=w320:errorcluster)  [unwired: 1 out]
      }
      frame "Mouse speed" {
        n92 = property class="Ctl"(reference=w327, error in=w326, "Value"=waveform(dbl)[] [] ("History Data"), "DisabledEnum"=T26."Disabled and Grayed Out" ("Disabled")) -> (error out=w325:errorcluster)  [unwired: 1 out]
      }
      frame "Mouse speed, mm/s" {
        n93 = property class="Ctl"(reference=w332, error in=w331, "Value"=0.0, "DisabledEnum"=T26."Disabled and Grayed Out" ("Disabled")) -> (error out=w330:errorcluster)  [unwired: 1 out]
      }
      frame "Run distance, m", "Running, perc. of time" {
        n94 = property class="Ctl"(reference=w337, error in=w336, "Value"=0.0, "DisabledEnum"=T26."Disabled and Grayed Out" ("Disabled")) -> (error out=w335:errorcluster)  [unwired: 1 out]
      }
      frame "Reward and stimulation" {
        n95 = property class="Ctl"(reference=w341, error in=w340, "DisabledEnum"=T26."Enabled" ("Disabled")) -> (error out=w339:errorcluster)  [unwired: 1 out]
      }
      frame "Histograms" {
        w345 = refnum<vi> refnum  # XYGraph
        n96 = To More Specific Class(target class=w345, reference=w348, error in=w344) -> (specific class reference=w346:refnum<vi>, error out=w343:errorcluster)
        n97 = disable-structure shown="Disabled" {
          frame Disabled {
          }
          frame Enabled {
          }
        }
        n98 = property class="XYGraph"(reference=w346, error in=w343, "DisabledEnum"=T26."Disabled" ("Disabled")) -> (error out=w347:errorcluster)  [unwired: 1 out]
      }
      frame "Current zone" {
        w355 = refnum<vi> refnum  # Cluster
        n99 = To More Specific Class(target class=w355, reference=w350, error in=w352) -> (specific class reference=w353:refnum<vi>, error out=w354:errorcluster)
        n100 = call "UI_update_Zone_indicator_params_(univ).vi"("error in (no error)"=w354, "Geometry"=w351, "Zone indicator ref. in"=w353) -> ("error out"=w349:errorcluster)  [unwired: 7 in, 1 out]
      }
    }
    n101 = Build Array(w287, w286) -> (w285:string[])
  }
  "Indicators references params" <- w26
  n102 = call "SW_Get_Menu_tags.vi"("Menu ref in"=w4, "error in (no error)"=w3) -> ("Menu ref out"=w6:refnum<k9>, "(Sub)menu tags"=w8:string[], "error out"=w7:errorcluster)
  n103 = for {
    tunnel: w8 -> [w360] mode=indexing
    tunnel: w7 -> [w359]
    tunnel: [w358] -> w5 mode=indexing
    tunnel: [w357] -> _
    tunnel: w6 -> [w356]
    n104 = case shown="\"Fix broken track\"" w360 {
      selector: w360 -> [_ w368 w374 w380 w386 w392 w398 w404 w410 w416 w422]
      tunnel: w359 -> [w362 w366 w372 w378 w384 w390 w396 w402 w408 w414 w420]
      tunnel: [w362 w365 w371 w377 w383 w389 w395 w401 w407 w413 w419] -> w358
      tunnel: [w361 w364 w370 w376 w382 w388 w394 w400 w406 w412 w418] -> w357
      tunnel: w356 -> [w361 w363 w369 w375 w381 w387 w393 w399 w405 w411 w417]
      frame "", Default {
      }
      frame "Play Start" {
        n105 = Set Menu Item Info(7:w368, 8:w366, 9:TRUE ("enabled"), 11:w363) -> (0:w365:errorcluster, 3:w364:refnum<k9>)  [unwired: 3 in]
      }
      frame "Play Stop" {
        n106 = Set Menu Item Info(7:w374, 8:w372, 9:FALSE ("enabled"), 11:w369) -> (0:w371:errorcluster, 3:w370:refnum<k9>)  [unwired: 3 in]
      }
      frame "Fix broken track" {
        n107 = Set Menu Item Info(7:w380, 8:w378, 9:TRUE ("enabled"), 11:w375) -> (0:w377:errorcluster, 3:w376:refnum<k9>)  [unwired: 3 in]
      }
      frame "Tools" {
        n108 = Set Menu Item Info(7:w386, 8:w384, 9:TRUE ("enabled"), 11:w381) -> (0:w383:errorcluster, 3:w382:refnum<k9>)  [unwired: 3 in]
      }
      frame "I/O Configuration" {
        n109 = Set Menu Item Info(7:w392, 8:w390, 9:TRUE ("enabled"), 11:w387) -> (0:w389:errorcluster, 3:w388:refnum<k9>)  [unwired: 3 in]
      }
      frame "Cage and Recording" {
        n110 = Set Menu Item Info(7:w398, 8:w396, 9:TRUE ("enabled"), 11:w393) -> (0:w395:errorcluster, 3:w394:refnum<k9>)  [unwired: 3 in]
      }
      frame "Timings calibration" {
        n111 = Set Menu Item Info(7:w404, 8:w402, 9:TRUE ("enabled"), 11:w399) -> (0:w401:errorcluster, 3:w400:refnum<k9>)  [unwired: 3 in]
      }
      frame "Dispension rate calibration" {
        n112 = Set Menu Item Info(7:w410, 8:w408, 9:TRUE ("enabled"), 11:w405) -> (0:w407:errorcluster, 3:w406:refnum<k9>)  [unwired: 3 in]
      }
      frame "Save Settings" {
        n113 = Set Menu Item Info(7:w416, 8:w414, 9:TRUE ("enabled"), 11:w411) -> (0:w413:errorcluster, 3:w412:refnum<k9>)  [unwired: 3 in]
      }
      frame "Load Settings" {
        n114 = Set Menu Item Info(7:w422, 8:w420, 9:TRUE ("enabled"), 11:w417) -> (0:w419:errorcluster, 3:w418:refnum<k9>)  [unwired: 3 in]
      }
    }
  }
  n115 = Merge Errors(w5) -> (w2:errorcluster)
  n116 = Merge Errors(w2, w12, w18) -> (w17:errorcluster)
  n117 = property class="Pnl"(reference=w15, error in=w17, "DeferPanUpdts"=FALSE ("Defer Panel Updates")) -> (error out=→"error out":errorcluster)  [unwired: 1 out]
  "All references out" <- "All references in"
  "Settings cluster out" <- "Settings cluster in"
